vi "NI9210_TemperatureInputs_v2.vi"() -> ()   [LabVIEW 2025]
uses:
  <vilib>/DAQmx/read.llb/DAQmx Read (Analog 1D Wfm NChan NSamp).vi
  <vilib>/DAQmx/configure/timing.llb/DAQmx Timing (Sample Clock).vi
  <vilib>/DAQmx/miscellaneous.llb/DAQmx Fill In Error Info.vi
panel:
  out "error out":errorcluster
  out "TC3 - Supply Oxidizer Thermocouple":dynamicdata(graph)
  out "TC2 - Inlet Thermocouple":dynamicdata(graph)
  out "TC1 - Upstream Thermocouple":dynamicdata(graph)
  in  "stop":bool
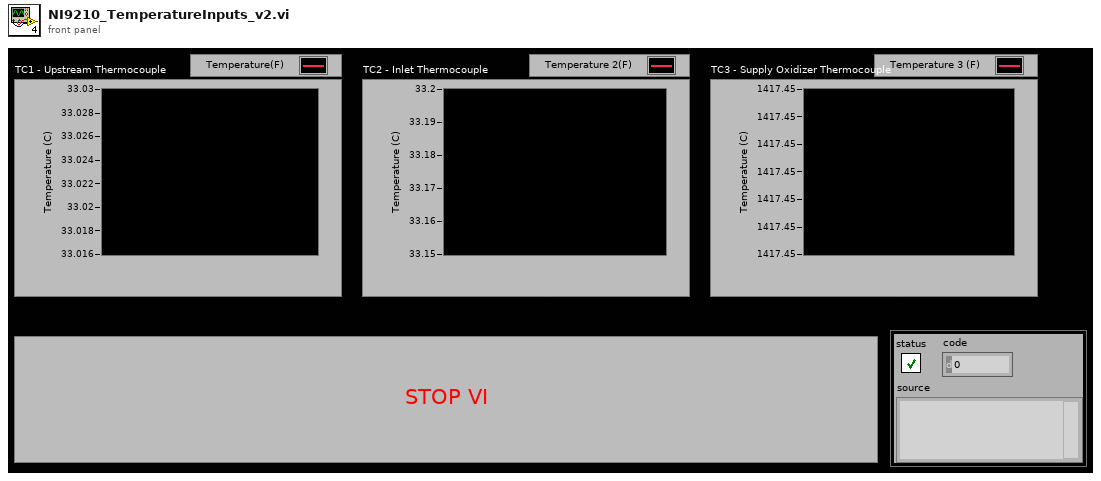
[diagram p1: front panel]
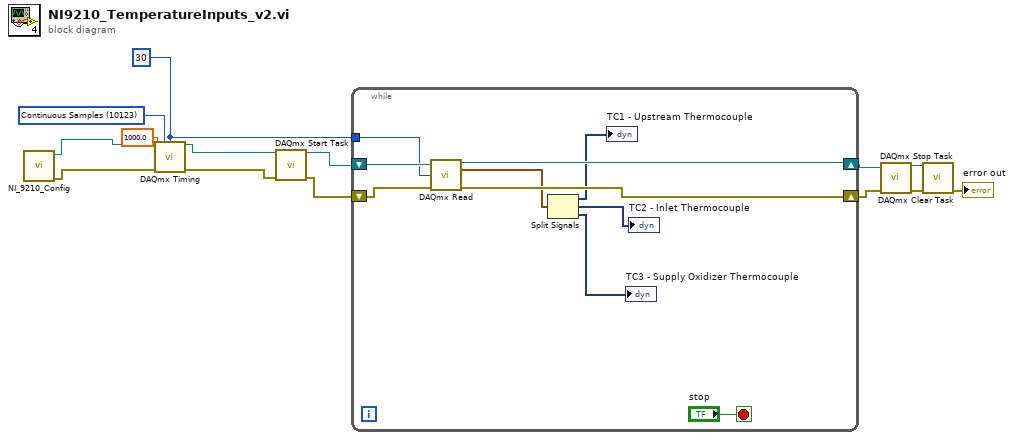
[diagram p0: block diagram]
diagram:
  w7 = 30 ("samples per channel")
  w12 = 10123 items=["Finite Samples"=10178, "Continuous Samples"=10123, "Hardware Timed Single Point"=12522] ("sample mode")
  n1 = call "NI_9210_Config.vi"() -> ("error out"=w13:errorcluster, "task out"=w14:refnum<k21>)  [unwired: 10 in]
  n2 = call-poly <vilib>:"DAQmx Timing.vi"("task/channels in"=w14, "sample mode"=w12, "samples per channel"=w7, "rate"=1000.0, "error in"=w13) -> ("task out"=w11:refnum<k21>, "error out"=w10:errorcluster)  [unwired: 9 in]
  n3 = call <vilib>:"DAQmx Start Task.vi"("task/channels in"=w11, "error in"=w10) -> ("task out"=w9:refnum<k21>, "error out"=w8:errorcluster)  [unwired: 12 in]
  n4 = while {
    shift-right: [w21] -> w3
    shift-left: w9 -> [w24]
    shift-right: [w20] -> w2
    shift-left: w8 -> [w23]
    tunnel: w7 -> [w22]
    stop <- "stop" stop-if-true
    n5 = call-poly <vilib>:"DAQmx Read.vi"("task/channels in"=w24, "number of samples per channel"=w22, "error in"=w23) -> ("task out"=w21:refnum<k21>, "data"=w19:waveform(dbl)[], "error out"=w20:errorcluster)  [unwired: 10 in]
    n6 = Split Signals(w19) -> (→"TC1 - Upstream Thermocouple":dynamicdata, →"TC2 - Inlet Thermocouple":dynamicdata, →"TC3 - Supply Oxidizer Thermocouple":dynamicdata)  [unwired: 3 in]
  }
  n7 = call <vilib>:"DAQmx Stop Task.vi"("task/channels in"=w3, "error in"=w2) -> ("task out"=w4:refnum<k21>, "error out"=w5:errorcluster)  [unwired: 12 in]
  n8 = call <vilib>:"DAQmx Clear Task.vi"("task in"=w4, "error in"=w5) -> ("error out"=→"error out":errorcluster)  [unwired: 13 in]
